vi "Home_Position.vi"(1 "Boolean":bool) -> ()   [LabVIEW 2013]
doc: "This subvi is intended to take the KOSY3 platform to the home position (0,0,0)"
panel:
  in  "Port for KOSY3":refnum<visa-resource-name>="COM2"
  out "Cordinates":T1 {"Schritte B" format="%#.4g"; "Schritte A" format="%#.4g"; "Schritte C" format="%#.4g"; "Schritte U" format="%#.4g"; "Schritte Z" format="%#.4g"; "Schritte Y" format="%#.4g"; "Schritte X" format="%#.4g"}
  out "error out":errorcluster
  in  "error in":errorcluster
  out "Stopped":bool
  out "Moving":bool
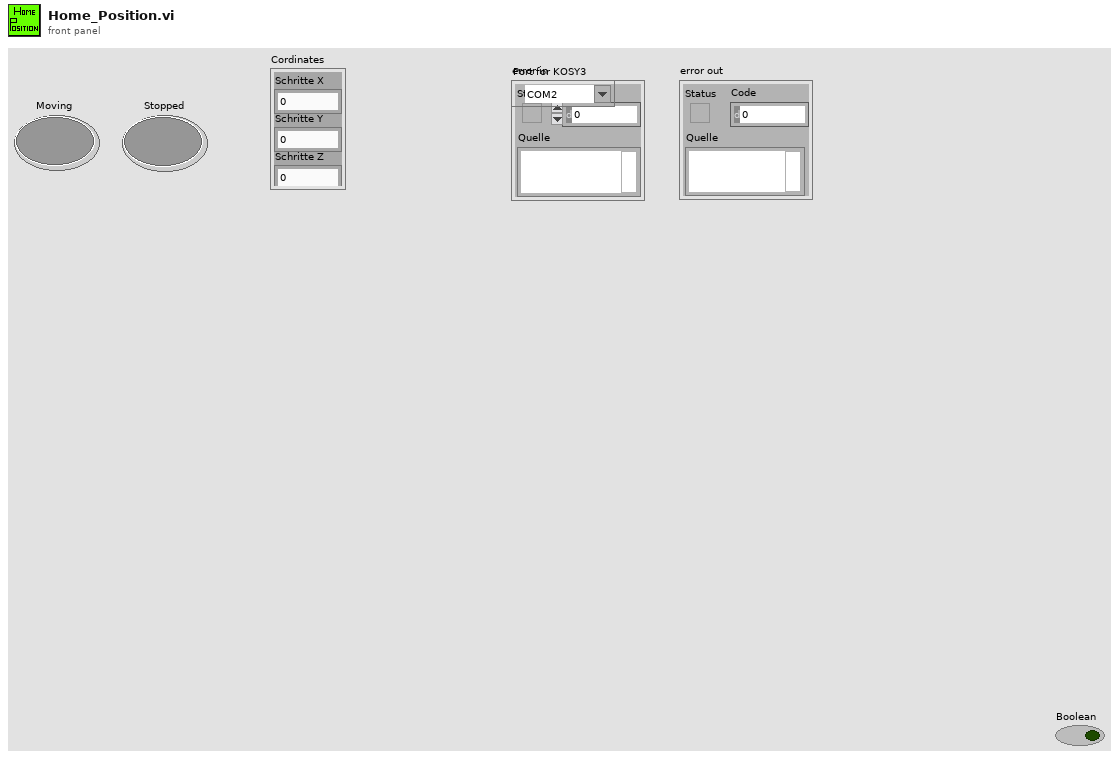
[diagram p1: front panel]
types:
  T1 = cluster{"Schritte X":sgl, "Schritte Y":sgl, "Schritte Z":sgl, "Schritte U":sgl, "Schritte C":sgl, "Schritte A":sgl, "Schritte B":sgl}
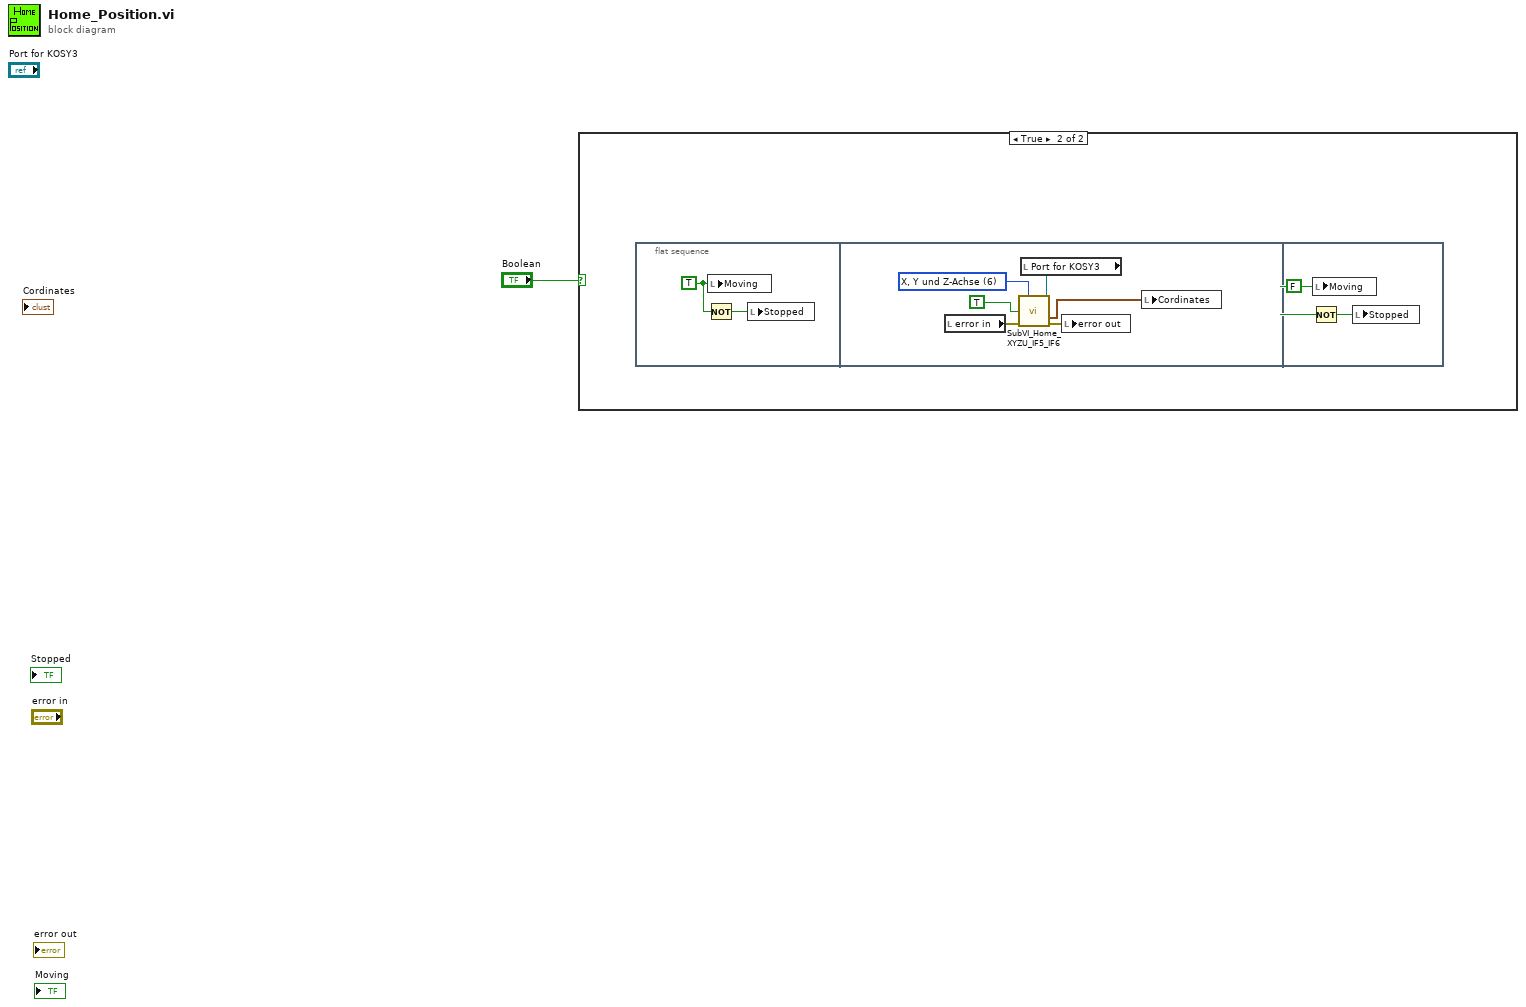
[diagram p0: block diagram]
diagram:
  n1 = case shown="True" "Boolean" {
    frame False {
    }
    frame True {
      n2 = flat-sequence {
        frame #0 {
          w2 = TRUE ("Moving")
          n3 = Not(x=w2) -> (.not. x?=w3:bool)
          n4 = local write "Moving"(w2) -> ()
          n5 = local write "Stopped"(w3) -> ()
        }
        frame #1 {
          w5 = u16 6 items=["X-Achse", "Y-Achse", "Z-Achse", "X- und Y-Achse", "X- und Z-Achse", "Y- und Z-Achse", "X, Y und Z-Achse", "U-Achse", "keine Achse"] ("Beteiligte Achsen (X,Y,Z,U)")
          n6 = local read "error in"() -> (w6:errorcluster)
          n7 = local read "Port for KOSY3"() -> (w8:refnum<visa-resource-name>)
          n8 = call "SubVI_Home_XYZU_IF5_IF6.vi"("VISA resource name in"=w8, "Beteiligte Achsen (X,Y,Z,U)"=w5, "IF5=F/IF6=T\n(IF6=T) in"=TRUE ("IF5=F/IF6=T\n(IF6=T) in"), "error in"=w6) -> ("Koordinaten IF6"=w4:T1, "error out"=w7:errorcluster)  [unwired: 4 in, 6 out]
          n9 = local write "error out"(w7) -> ()
          n10 = local write "Cordinates"(w4) -> ()
        }
        frame #2 {
          w10 = FALSE ("Moving")
          n11 = Not(x=w10) -> (.not. x?=w11:bool)
          n12 = local write "Moving"(w10) -> ()
          n13 = local write "Stopped"(w11) -> ()
        }
      }
    }
  }
